vi "multiswitch.vi"() -> ()   [LabVIEW 2012]
uses:
  Type Defs/4 Way Button.ctl
panel:
  out "x = y? 2":T1
  out "x = y?":bool[](array[boolean])
  in  "Mode Select":enum8{"Off", "Stby", "Hold", "Run"}(ring)
  in  "Mode 3":T1
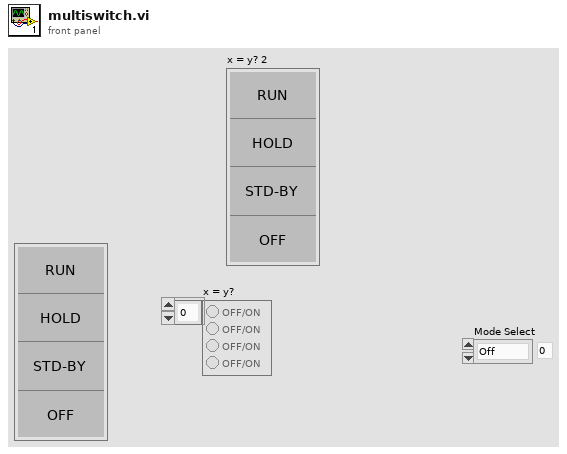
[diagram p1: front panel]
types:
  T1 = typedef "4 Way Button.ctl" = cluster{"Off":bool, "Standby":bool, "Hold":bool, "Run":bool}
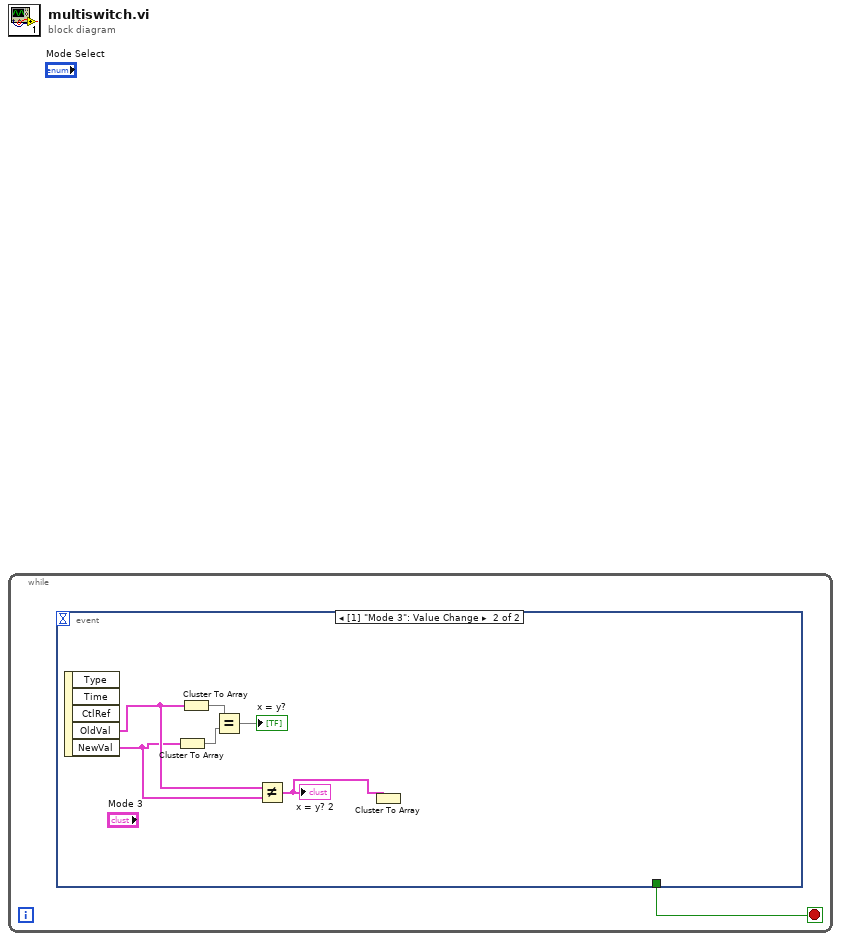
[diagram p0: block diagram]
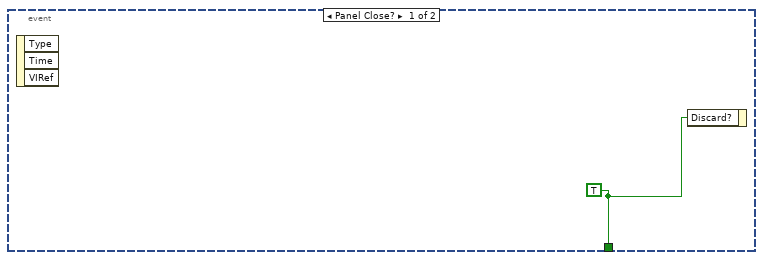
[diagram p2: hidden frame]
diagram:
  n1 = while {
    stop <- w1 stop-if-true
    n2 = event shown="[1] \"Mode 3\": Value Change" {
      selector: _ -> [_ _]
      dyn-events: _ -> [_ _]
      timeout: _ -> [_ _]
      tunnel: [w2 _] -> w1
      event Panel Close? {
        w2 = TRUE
        n3 = event-data() -> ()  [unwired: 1 in, 3 out]
        n4 = event-data("Discard?"=w2) -> ()  [unwired: 1 in, 1 out]
      }
      event Value Change {
        n5 = event-data() -> ("OldVal"=w5:T1, "NewVal"=w4:T1)  [unwired: 1 in, 3 out]
        n6 = Cluster To Array(cluster=w4) -> (array=w8:bool[])
        n7 = Cluster To Array(cluster=w5) -> (array=w7:bool[])
        n8 = Equal?(x=w7, y=w8) -> (x = y?=→"x = y?":bool[])
        n9 = Not Equal?(x=w5, y=w4) -> (x != y?=w3:T1)
        "x = y? 2" <- w3
        n10 = Cluster To Array(cluster=w3) -> ()  [unwired: 1 out]
      }
    }
  }
